vi "avgTable.vi"(0 "Data in":T1, 5 "Avg Voltage":dbl, 7 "Avg Current":dbl, 9 "Avg Resistance":dbl, 11 "Avg Temperature":dbl, 12 "u_A(temp)":dbl, 13 "Timestamp string":string[](array[string])) -> (4 "Data out":T1, 15 "Table":string[][](array[string]))   [LabVIEW 2022 SP3]
uses:
  controls/Data.ctl
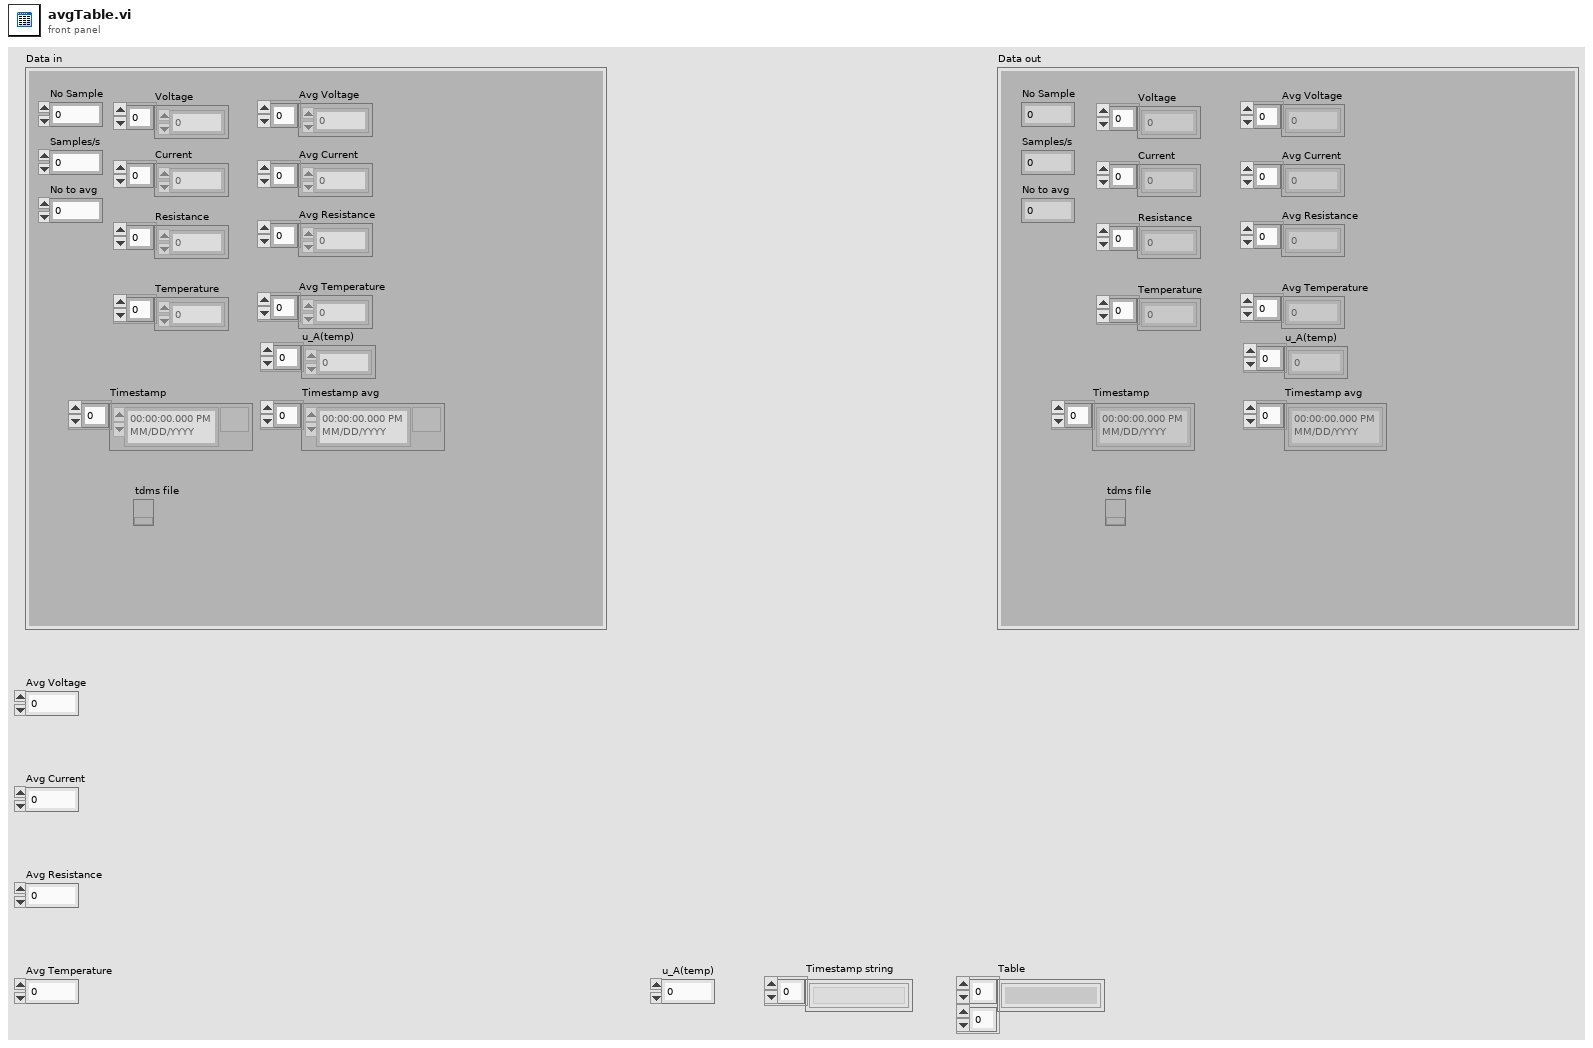
[diagram p1: front panel]
types:
  T1 = typedef "Data.ctl" = cluster{"No Sample":u16, "Samples/s":u16, "No to avg":u16, "Voltage":dbl[], "Current":dbl[], "Resistance":dbl[], "Temperature":dbl[], "Avg Voltage":dbl[], "Timestamp":timestamp[], "Avg Current":dbl[], "tdms file":refnum<k34>, "Timestamp avg":timestamp[], "Avg Resistance":dbl[], "Avg Temperature":dbl[], "u_A(temp)":dbl[]}
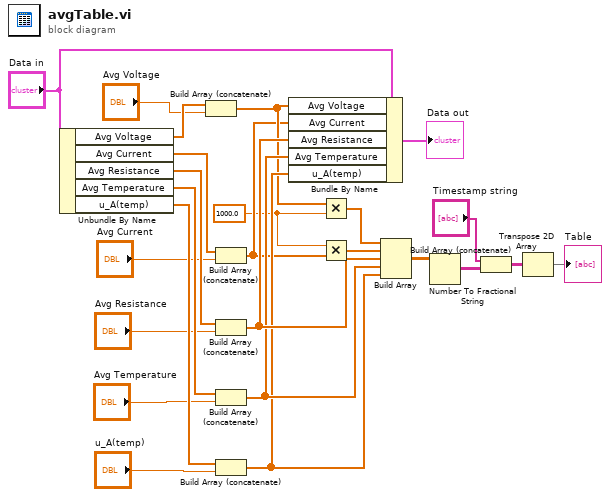
[diagram p0: block diagram]
diagram:
  w1 = 1000.0 ("Avg Voltage")
  n1 = Unbundle By Name("Data in") -> ("Avg Voltage"=w25:dbl[], "Avg Current"=w24:dbl[], "Avg Resistance"=w23:dbl[], "Avg Temperature"=w22:dbl[], "u_A(temp)"=w21:dbl[])
  n2 = Build Array (concatenate)(w25, "Avg Voltage") -> (w5:dbl[])
  n3 = Build Array (concatenate)(w24, "Avg Current") -> (w2:dbl[])
  n4 = Build Array (concatenate)(w23, "Avg Resistance") -> (w13:dbl[])
  n5 = Build Array (concatenate)(w22, "Avg Temperature") -> (w12:dbl[])
  n6 = Build Array (concatenate)(w21, "u_A(temp)") -> (w11:dbl[])
  n7 = Bundle By Name(cluster="Data in", "Avg Voltage"=w5, "Avg Current"=w2, "Avg Resistance"=w13, "Avg Temperature"=w12, "u_A(temp)"=w11) -> (→"Data out":T1)
  n8 = Multiply(x=w5, y=w1) -> (x*y=w4:dbl[])
  n9 = Multiply(x=w1, y=w2) -> (x*y=w3:dbl[])
  n10 = Build Array(w4, w3, w13, w12, w11) -> (w10:dbl[][])
  n11 = Number To Fractional String(number=w10) -> (F-format string=w9:string[][])  [unwired: 3 in]
  n12 = Build Array (concatenate)("Timestamp string", w9) -> (w7:string[][])
  n13 = Transpose 2D Array(2D array=w7) -> (transposed array=→"Table":string[][])
